vi "Exit.vi"(8 "Error In":errorcluster) -> (0 "Error Out":errorcluster)   [LabVIEW 2023, in "QSM - IODocs.lvlib"]
doc: "This VI sends the Exit message to the Queued Message Handler template."
uses:
  QSM - IODocs.lvlib
  Controls/Message Queue Element Position.ctl
  SubVIs/Enqueue Message (Single).vi
  Controls/State Machine Message.ctl
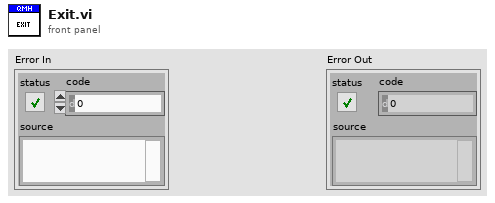
[diagram p1: front panel]
types:
  T1 = typedef "QSM - IODocs.lvlib/State Machine Message.ctl" = enum16{"Initialize", "BIAS ZERO", "DIFF ZERO", "DIFF TOGGLE", "Handle Error", "Exit"}
  T2 = typedef "QSM - IODocs.lvlib/Message Queue Element Position.ctl" = enum16{"Front", "Back"}
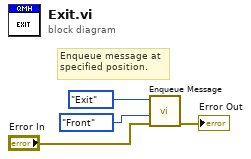
[diagram p0: block diagram]
diagram:
  # "Enqueue message at\nspecified position."
  n1 = call-poly "Enqueue Message.vi"("Error In"="Error In", "Message Position"=Message_Queue_Element_Position."Front", "State Machine Message"=State_Machine_Message."Exit") -> ("Error Out"=→"Error Out":errorcluster)  [unwired: 8 in]
